vi "4155C Config I Stress v3.0.vi"(3 "Stress I - Drain/Gate":u32(ring)=1 items=["SMU1  ", "SMU2  ", "SMU3  ", "SMU4  ", "SMU5  ", "SMU6  ", "VSU1  ", "VSU2  "], 4 "Stress I - Source/Common":u32(ring) items=["SMU1  ", "SMU2  ", "SMU3  ", "SMU4  ", "SMU5  ", "SMU6  ", "VSU1  ", "VSU2  "], 5 "Display on/off":bool, 6 "error in (no error)":errorcluster, 7 "VDG compliance":dbl min=0.0 max=100000000000.0 format="%.15e", 8 "IDG":dbl min=0.0 max=100000000000.0 format="%.15e", 9 "VISA session":refnum<visa-resource-name>) -> (0 "error out":errorcluster, 2 "dup VISA resource name":refnum<visa-resource-name>)   [LabVIEW 2016]
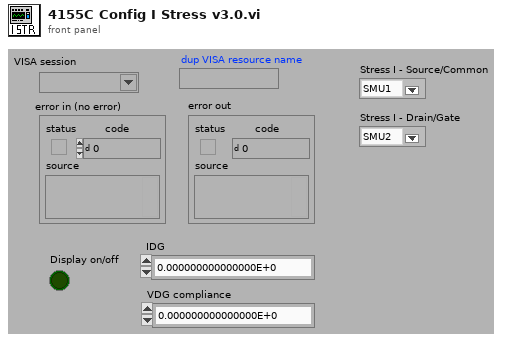
[diagram p1: front panel]
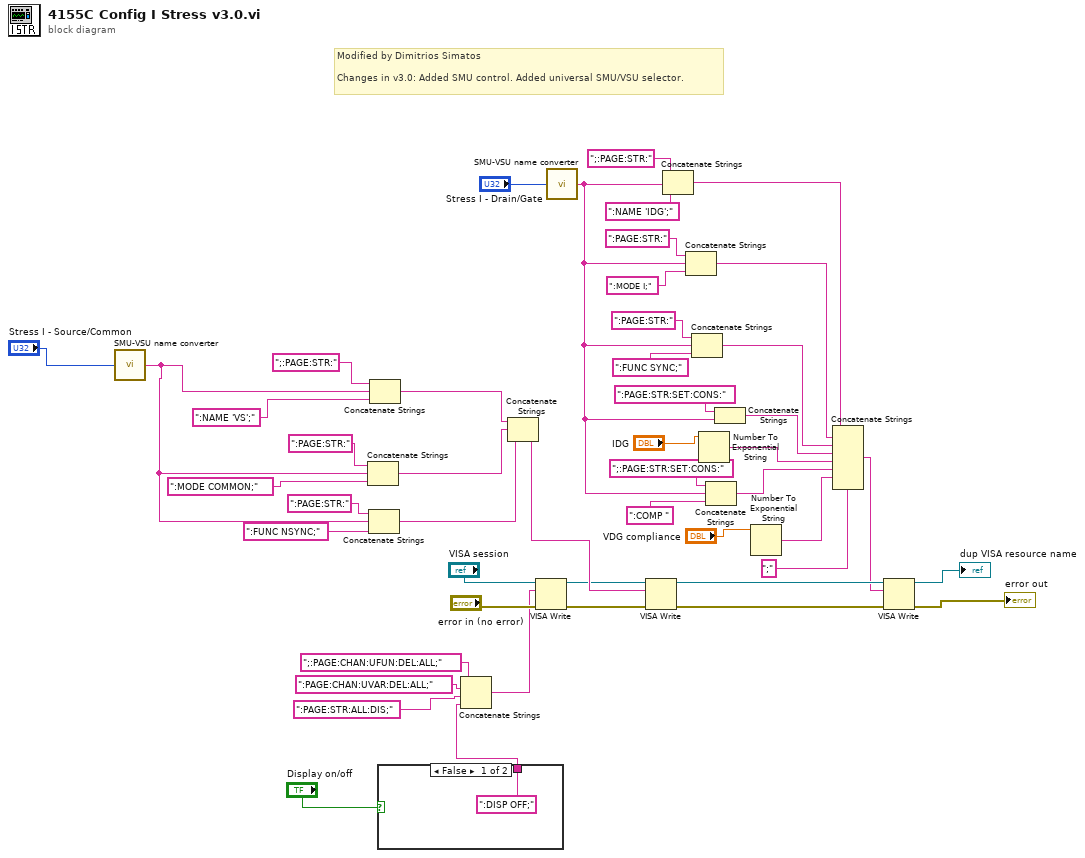
[diagram p0: block diagram]
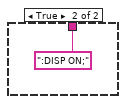
[diagram p2: hidden frame]
diagram:
  # "Modified by Dimitrios Simatos\n\nChanges in v3.0: Added SMU control. Added universal SMU/VSU selector."
  n1 = call "SMU-VSU name converter.vi"("unit to configure"="Stress I - Source/Common") -> ("SMU/VSU to be configured"=w22:string)
  n2 = Concatenate Strings(":PAGE:STR:", w22, ":MODE COMMON;") -> (w23:string)
  n3 = Concatenate Strings(":PAGE:STR:", w22, ":FUNC NSYNC;") -> (w21:string)
  n4 = Concatenate Strings(";:PAGE:STR:", w22, ":NAME 'VS';") -> (w27:string)
  n5 = case shown="False" "Display on/off" {
    tunnel: [":DISP OFF;" ("write buffer (\"\")") ":DISP ON;" ("write buffer (\"\")")] -> w42
    frame False {
    }
    frame True {
    }
  }
  n6 = Concatenate Strings(";:PAGE:CHAN:UFUN:DEL:ALL;", ":PAGE:CHAN:UVAR:DEL:ALL;", ":PAGE:STR:ALL:DIS;", w42) -> (w43:string)
  n7 = Concatenate Strings(w27, w23, w21) -> (w33:string)
  n8 = VISA Write(VISA resource name="VISA session", write buffer=w43, error in (no error)="error in (no error)") -> (VISA resource name out=w32:refnum<visa-resource-name>, error out=w31:errorcluster)  [unwired: 1 out]
  n9 = call "SMU-VSU name converter.vi"("unit to configure"="Stress I - Drain/Gate") -> ("SMU/VSU to be configured"=w1:string)
  n10 = VISA Write(VISA resource name=w32, write buffer=w33, error in (no error)=w31) -> (VISA resource name out=w48:refnum<visa-resource-name>, error out=w47:errorcluster)  [unwired: 1 out]
  n11 = Concatenate Strings(";:PAGE:STR:", w1, ":NAME 'IDG';") -> (w13:string)
  n12 = Concatenate Strings(":PAGE:STR:", w1, ":MODE I;") -> (w10:string)
  n13 = Concatenate Strings(":PAGE:STR:", w1, ":FUNC SYNC;") -> (w7:string)
  n14 = Number To Exponential String(number="IDG") -> (E-format string=w36:string)  [unwired: 3 in]
  n15 = Concatenate Strings(";:PAGE:STR:SET:CONS:", w1, ":COMP ") -> (w2:string)
  n16 = Concatenate Strings(":PAGE:STR:SET:CONS:", w1) -> (w5:string)
  n17 = Number To Exponential String(number="VDG compliance") -> (E-format string=w34:string)  [unwired: 3 in]
  n18 = Concatenate Strings(w13, w10, w7, w5, w36, w2, w34, ";" ("Substring")) -> (w30:string)
  n19 = VISA Write(VISA resource name=w48, write buffer=w30, error in (no error)=w47) -> (VISA resource name out=→"dup VISA resource name":refnum<visa-resource-name>, error out=→"error out":errorcluster)  [unwired: 1 out]
